vi "IB_RW_Project_DistPart.vi"(7 "action":T3, 8 "error in (no error)":errorcluster, 9 "index in":string, 10 "DistParts":T2, 11 "buildObject":T1) -> (0 "error out":errorcluster, 1 "index out":string, 2 "DistParts":T2, 3 "buildObject out":T1)   [LabVIEW 2020]
doc: "Reads and writes the data to the object property bag."
uses:
  <resource>/Framework/Providers/API/ItemRef.ctl
  <vilib>/AppBuilder/IB_RW_Project/IB_RW_Project_DistPart_Data.ctl
  <vilib>/AppBuilder/IB_RW_Project/IB_RW_Project_PropBag_Action.ctl
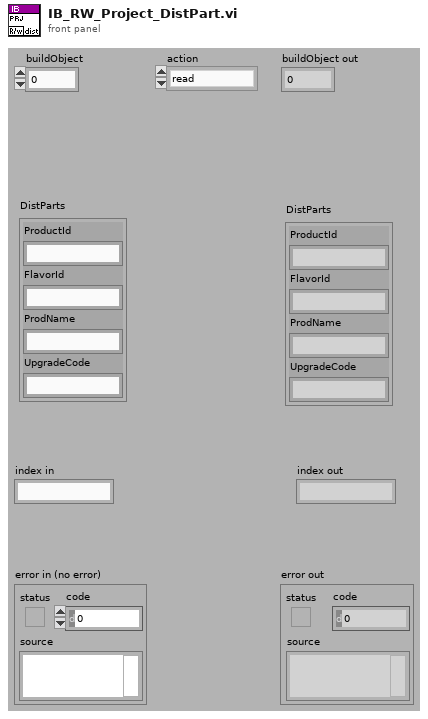
[diagram p1: front panel]
types:
  T1 = typedef "ItemRef.ctl" = u64
  T2 = typedef "IB_RW_Project_DistPart_Data.ctl" = cluster{"ProductId":string, "FlavorId":string, "ProdName":string, "UpgradeCode":string}
  T3 = typedef "IB_RW_Project_PropBag_Action.ctl" = enum16{"read", "write", "clear", "readPrevious", "writePrevious", "clearPrevious"}
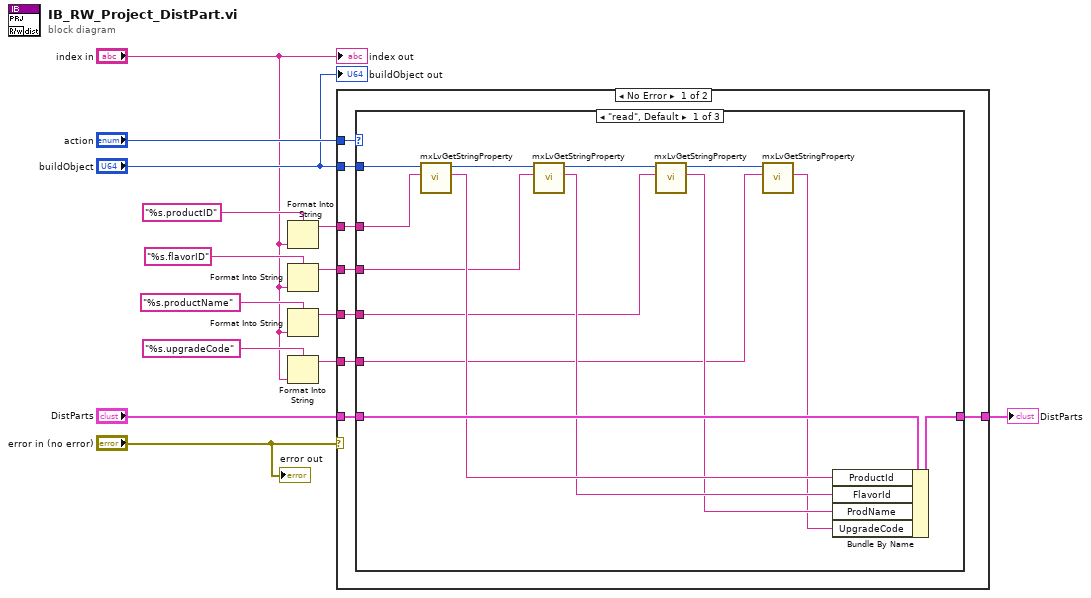
[diagram p0: block diagram]
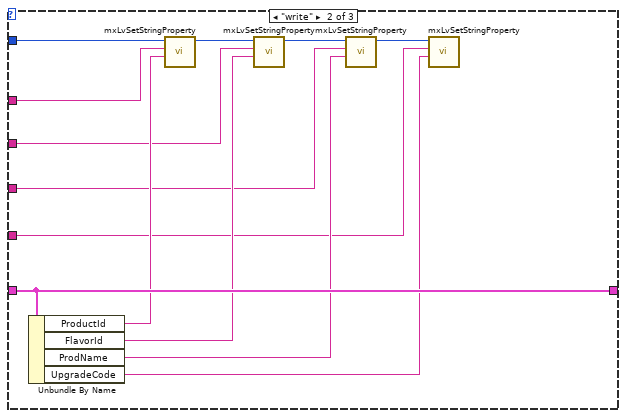
[diagram p2: hidden frame]
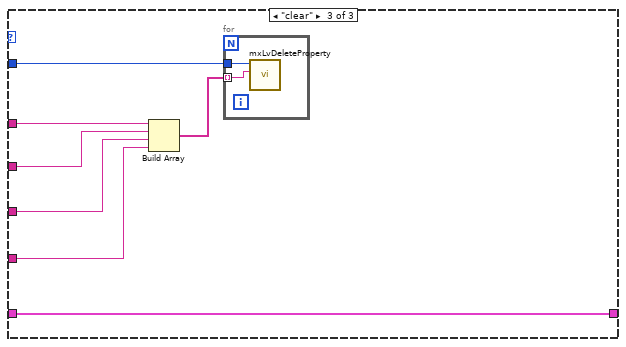
[diagram p3: hidden frame]
diagram:
  n1 = Format Into String(format string="%s.productID", "index in") -> (resulting string=w11:string)  [unwired: 2 in, 1 out]
  n2 = Format Into String(format string="%s.flavorID", "index in") -> (resulting string=w6:string)  [unwired: 2 in, 1 out]
  n3 = Format Into String(format string="%s.productName", "index in") -> (resulting string=w4:string)  [unwired: 2 in, 1 out]
  n4 = Format Into String(format string="%s.upgradeCode", "index in") -> (resulting string=w2:string)  [unwired: 2 in, 1 out]
  n5 = case shown="No Error" "error in (no error)" {
    tunnel: "action" -> [w22 _]
    tunnel: "DistParts" -> [w21 w59]
    tunnel: w11 -> [w20 _]
    tunnel: w4 -> [w19 _]
    tunnel: [w18 w59] -> w10
    tunnel: "buildObject" -> [w17 _]
    tunnel: w6 -> [w16 _]
    tunnel: w2 -> [w15 _]
    frame No Error {
      n6 = case shown="\"read\", Default" w22 {
        tunnel: w17 -> [w34 w48 w50]
        tunnel: w21 -> [w36 w49 w56]
        tunnel: w20 -> [w32 w45 w55]
        tunnel: w19 -> [w27 w41 w53]
        tunnel: [w35 w49 w56] -> w18
        tunnel: w16 -> [w30 w43 w54]
        tunnel: w15 -> [w24 w39 w52]
        frame "read", Default {
          n7 = call <resource>:"mxLvGetStringProperty.vi"("Tag"=w32, "Item"=w34) -> ("Value"=w31:string, "Item"=w33:T1)  [unwired: 1 in, 7 out]
          n8 = call <resource>:"mxLvGetStringProperty.vi"("Tag"=w30, "Item"=w33) -> ("Value"=w29:string, "Item"=w26:T1)  [unwired: 1 in, 7 out]
          n9 = call <resource>:"mxLvGetStringProperty.vi"("Tag"=w27, "Item"=w26) -> ("Value"=w28:string, "Item"=w25:T1)  [unwired: 1 in, 7 out]
          n10 = call <resource>:"mxLvGetStringProperty.vi"("Tag"=w24, "Item"=w25) -> ("Value"=w23:string)  [unwired: 1 in, 8 out]
          n11 = Bundle By Name(cluster=w36, "ProductId"=w31, "FlavorId"=w29, "ProdName"=w28, "UpgradeCode"=w23) -> (w35:T2)
        }
        frame "write" {
          n12 = Unbundle By Name(w49) -> ("ProductId"=w44:string, "FlavorId"=w42:string, "ProdName"=w40:string, "UpgradeCode"=w37:string)
          n13 = call <resource>:"mxLvSetStringProperty.vi"("Value (\"\")"=w44, "Tag"=w45, "Item"=w48) -> ("Item"=w47:T1)  [unwired: 2 in, 6 out]
          n14 = call <resource>:"mxLvSetStringProperty.vi"("Value (\"\")"=w42, "Tag"=w43, "Item"=w47) -> ("Item"=w46:T1)  [unwired: 2 in, 6 out]
          n15 = call <resource>:"mxLvSetStringProperty.vi"("Value (\"\")"=w40, "Tag"=w41, "Item"=w46) -> ("Item"=w38:T1)  [unwired: 2 in, 6 out]
          n16 = call <resource>:"mxLvSetStringProperty.vi"("Value (\"\")"=w37, "Tag"=w39, "Item"=w38) -> ()  [unwired: 2 in, 7 out]
        }
        frame "clear" {
          n17 = Build Array(w55, w54, w53, w52) -> (w51:string[])
          n18 = for {
            tunnel: w51 -> [w58] mode=indexing
            tunnel: w50 -> [w57]
            n19 = call <resource>:"mxLvDeleteProperty.vi"("Tag"=w58, "Item"=w57) -> ()  [unwired: 1 in, 9 out]
          }
        }
      }
    }
    frame Error {
    }
  }
  "DistParts" <- w10
  "error out" <- "error in (no error)"
  "buildObject out" <- "buildObject"
  "index out" <- "index in"
